vi "QCA - DUT Begin Receive.vi"(0 "CART TCP Connection In":refnum<k5>, 7 "Receive Config":T2={"Frequency, MHz"=2412, "Data Rate"="1,0,0", "Packet Count"=0, "RX Mac Address"="10:11:11:11:11:01", "TX Mac Address"="10:11:11:11:11:01", "BS Mac Address"="10:11:11:11:11:01", "Packet Length"=1000, "Broadcast"=FALSE}, 11 "error in (no error)":errorcluster) -> (4 "CART TCP Connection Out":refnum<k5>, 6 "Messages Logged":string[](array[string]), 14 "Command Sent":string, 15 "error out":errorcluster)   [LabVIEW 2011, in "ART2 Test Panel.lvlib"]
uses:
  ART2/ART2 Test Panel.lvlib
  ART2 Test Panel/Components/ART2.llb/CART/Controls/Data Rates.ctl
  ART2/SubVIs/NART Constants.vi
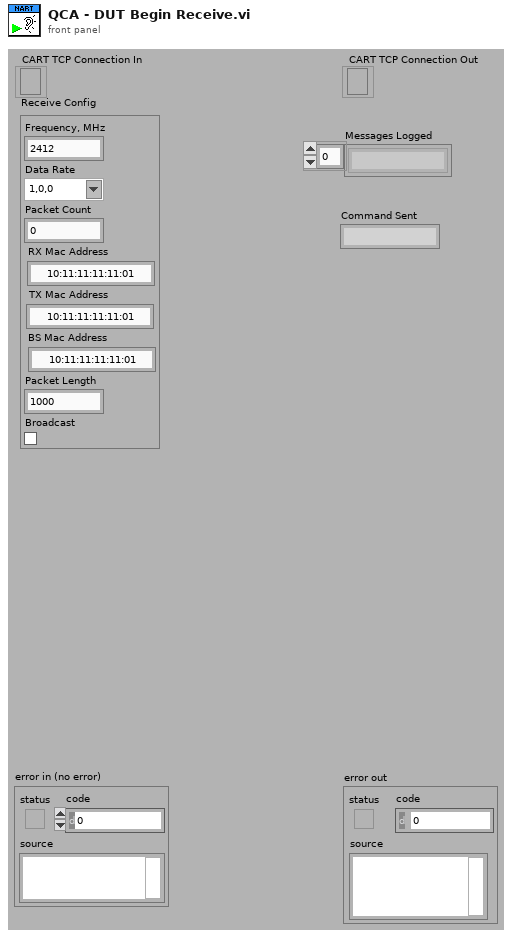
[diagram p1: front panel]
types:
  T1 = typedef "ART2 Test Panel.lvlib/Data Rates.ctl" = string
  T2 = cluster{"Frequency, MHz":u32, "Data Rate":T1, "Packet Count":i32, "RX Mac Address":string, "TX Mac Address":string, "BS Mac Address":string, "Packet Length":u32, "Broadcast":bool}
  T3 = cluster{"Name":string, "Type":enum16{"decimal", "string", "float", "hex"}}[]
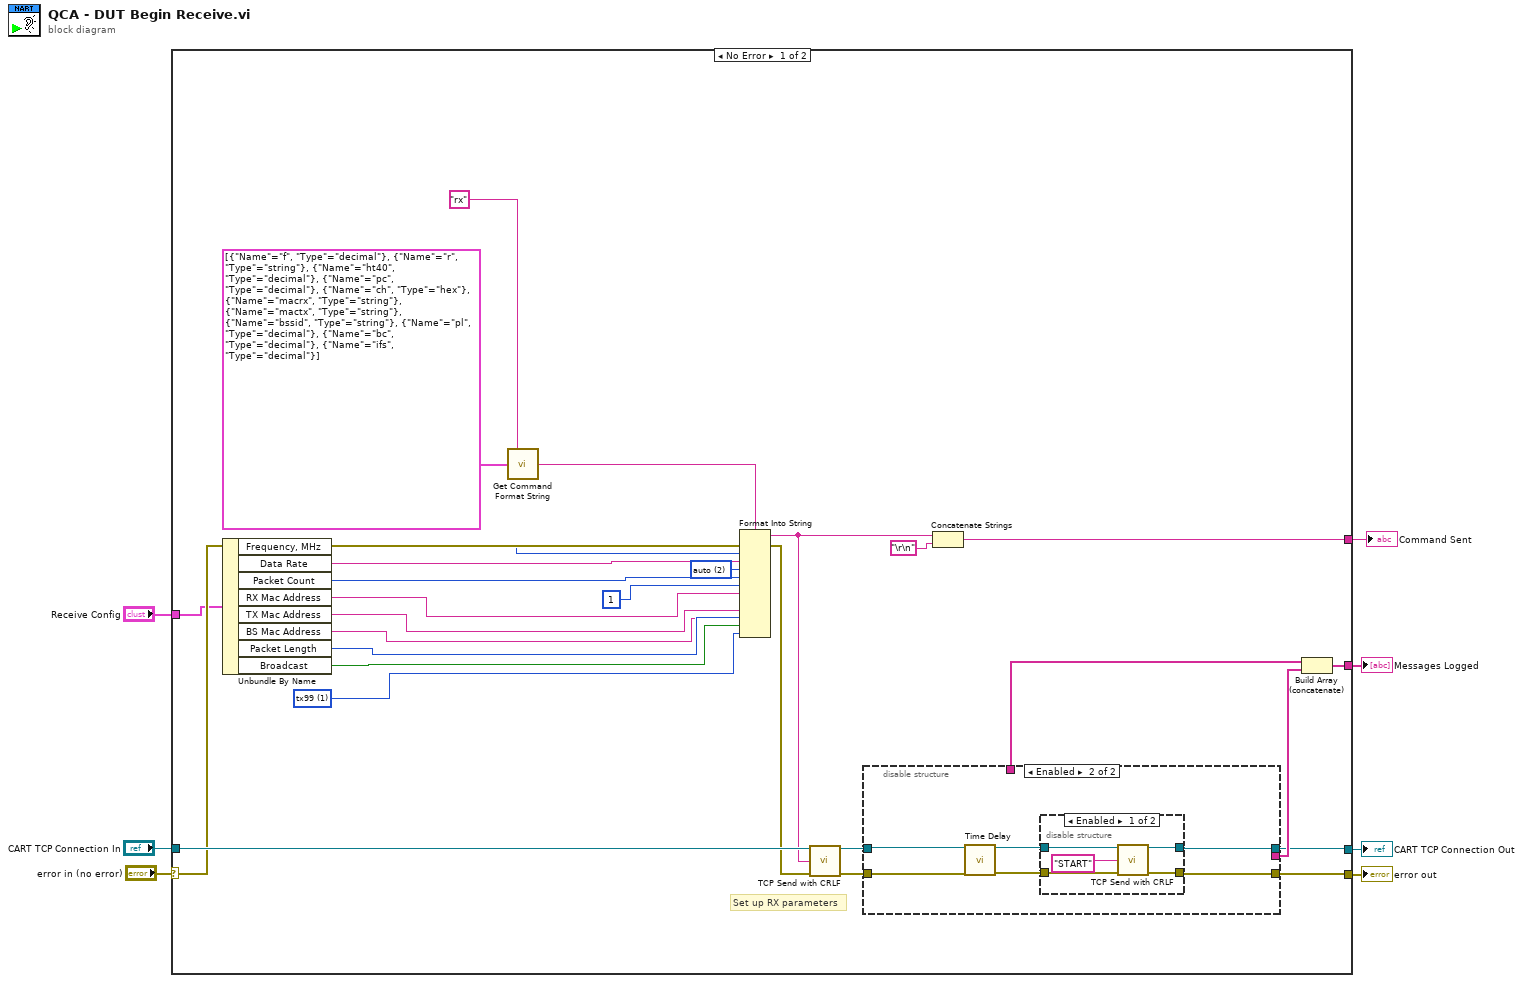
[diagram p0: block diagram]
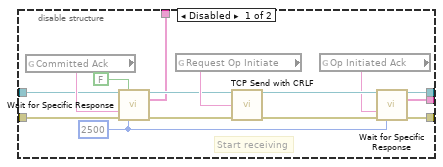
[diagram p2: hidden frame]
diagram:
  n1 = case shown="No Error" "error in (no error)" {
    selector: "error in (no error)" -> [w32 w64]
    tunnel: [w24 w64] -> w6
    tunnel: "CART TCP Connection In" -> [w35 w63]
    tunnel: [w23 w63] -> w4
    tunnel: "Receive Config" -> [w30 _]
    tunnel: [w27 _] -> w2
    tunnel: [w15 _] -> w1
    frame No Error {
      w8 = i16 1 items=["Regular"=-1, "tx100"=0, "tx99"=1] ("Inter Frame Spacing")
      w10 = i16 2 items=["none"=0, "low"=-1, "high"=1, "auto"=2] ("input 3")
      # "Set up RX parameters"
      n2 = Unbundle By Name(w30) -> ("Frequency, MHz"=w28:u32, "Data Rate"=w11:T1, "Packet Count"=w20:i32, "RX Mac Address"=w19:string, "TX Mac Address"=w18:string, "BS Mac Address"=w13:string, "Packet Length"=w17:u32, "Broadcast"=w12:bool)
      n3 = call "Get Command Format String.vi"("Command"="rx", "Parameters"=T3 [{"Name"="f", "Type"=enum."decimal"}, {"Name"="r", "Type"=enum."string"}, {"Name"="ht40", "Type"=enum."decimal"}, {"Name"="pc", "Type"=enum."decimal"}, {"Name"="ch", "Type"=enum."hex"}, {"Name"="macrx", "Type"=enum."string"}, {"Name"="mactx", "Type"=enum."string"}, {"Name"="bssid", "Type"=enum."string"}, {"Name"="pl", "Type"=enum."decimal"}, {"Name"="bc", "Type"=enum."decimal"}, {"Name"="ifs", "Type"=enum."decimal"}]) -> ("Command Format String"=w29:string)  [unwired: 13 in]
      n4 = Format Into String(format string=w29, error in=w32, w28, w11, w10, w20, 1 ("Chains"), w19, w18, w13, w17, w12, w8) -> (resulting string=w14:string, error out=w31:errorcluster)  [unwired: 1 in]
      n5 = call "TCP Send with CRLF.vi"("CART TCP Connection"=w35, "data in"=w14, "error IO"=w31) -> ("CART TCP Connection Out"=w22:refnum<k5>, "error out"=w21:errorcluster)  [unwired: 11 in]
      n6 = disable-structure shown="Enabled" {
        disable-tunnel: [w42 _] -> w26
        disable-tunnel: [w41 _] -> w25
        disable-tunnel: [w40 w53] -> w24
        disable-tunnel: [w39 w52] -> w23
        disable-tunnel: w22 -> [w38 w51]
        disable-tunnel: w21 -> [w37 w54]
        frame Disabled {
          w50 = 2500 ("Timeout (100ms)")
          # "Start receiving"
          n7 = global read "NART Constants.vi" "Committed Ack"() -> (w49:string)
          n8 = call "Wait for Specific Response.vi"("TCP Connection In"=w38, "Next response (t)"=FALSE, "Expected Message Start (\"\":any)"=w49, "error in"=w37, "Timeout (250 ms)"=w50) -> ("TCP Connection Out"=w46:refnum<k5>, "TCP Messages"=w42:string[], "error out"=w47:errorcluster)  [unwired: 7 in, 1 out]
          n9 = global read "NART Constants.vi" "Request Op Initiate"() -> (w48:string)
          n10 = call "TCP Send with CRLF.vi"("CART TCP Connection"=w46, "data in"=w48, "error IO"=w47) -> ("CART TCP Connection Out"=w45:refnum<k5>, "error out"=w43:errorcluster)  [unwired: 11 in]
          n11 = global read "NART Constants.vi" "Op Initiated Ack"() -> (w44:string)
          n12 = call "Wait for Specific Response.vi"("TCP Connection In"=w45, "Expected Message Start (\"\":any)"=w44, "error in"=w43, "Timeout (250 ms)"=w50) -> ("TCP Connection Out"=w39:refnum<k5>, "TCP Messages"=w41:string[], "error out"=w40:errorcluster)  [unwired: 8 in, 1 out]
        }
        frame Enabled {
          n13 = call "Time Delay"("error in (no error)"=w54) -> ("error out"=w55:errorcluster)  [unwired: 10 in]
          n14 = disable-structure shown="Enabled" {
            disable-tunnel: w51 -> [w60 w62]
            disable-tunnel: [w59 w61] -> w53
            disable-tunnel: [w58 w62] -> w52
            disable-tunnel: w55 -> [w57 w61]
            frame Enabled {
              n15 = call "TCP Send with CRLF.vi"("CART TCP Connection"=w60, "data in"="START" ("format string"), "error IO"=w57) -> ("CART TCP Connection Out"=w58:refnum<k5>, "error out"=w59:errorcluster)  [unwired: 11 in]
            }
            frame Disabled {
            }
          }
        }
      }
      n16 = Concatenate Strings(w14, "\r\n") -> (w15:string)
      n17 = Build Array (concatenate)(w26, w25) -> (w27:string[])
    }
    frame Error {
    }
  }
  "error out" <- w6
  "CART TCP Connection Out" <- w4
  "Messages Logged" <- w2
  "Command Sent" <- w1
